vi "Check_Position_PN.vi"(0 "Visualisation only (no collision detection)":bool, 4 "Extrusion mode":bool, 5 "Collision mode":T1=enum."Traverse - All", 6 "Model Rotation (deg)":sgl[](array[numeric])=[0.0, 0.0, 0.0] format="%.2g", 7 "Traverse extruded position":sgl[](array[numeric])=[0.0, 0.0, 0.0] format="%.2g", 8 "Position to check":sgl[](array[numeric])=[0.0, 0.0, 0.0] format="%.2g", 9 "Traverse Name":string) -> (1 "Collision":bool, 3 "Error Comments":string)   [LabVIEW 2016]
uses:
  Collision_Detection/Triangles/EnFlo specific/Collision Mode.ctl
  <vilib>/Analysis/coordinate.llb/Euler Rotation Order.ctl
  <vilib>/Analysis/coordinate.llb/3D Cartesian Coordinate Rotation (Euler) (Scalar).vi
  <vilib>/Analysis/baseanly.llb/Unit Vector (DBL).vi
  <vilib>/Analysis/baseanly.llb/Real Dot Product.vi
  Globals/Constants_global.vi
  <vilib>/Analysis/NI_AALPro.lvlib
  <vilib>/Analysis/NI_AALBase.lvlib
panel:
  in  "3D graphics output":bool=TRUE
  # "X\n\nY\n\nZ"
  # "Roll\n\nPitch\n\nYaw"
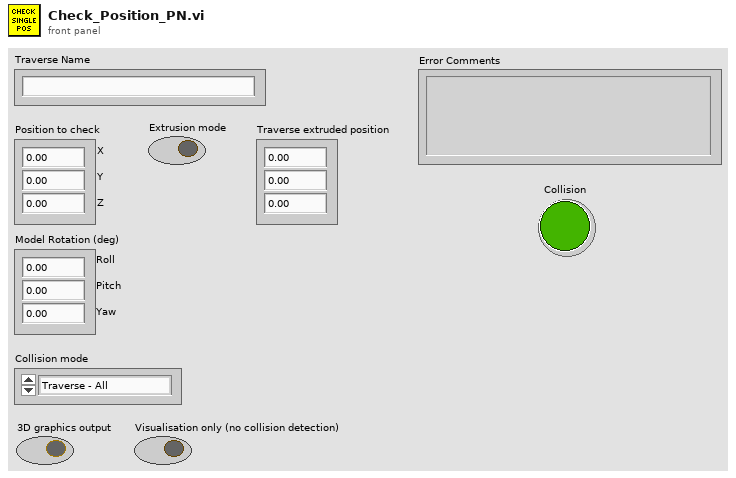
[diagram p1: front panel]
types:
  T1 = typedef "Collision Mode.ctl" = enum16{"Traverse - Tunnel", "Traverse - Model", "Traverse - Fixed objects", "Traverse - Traverse", "Traverse - All"}
  T2 = typedef "NI_AALPro.lvlib/Euler Rotation Order.ctl" = u16
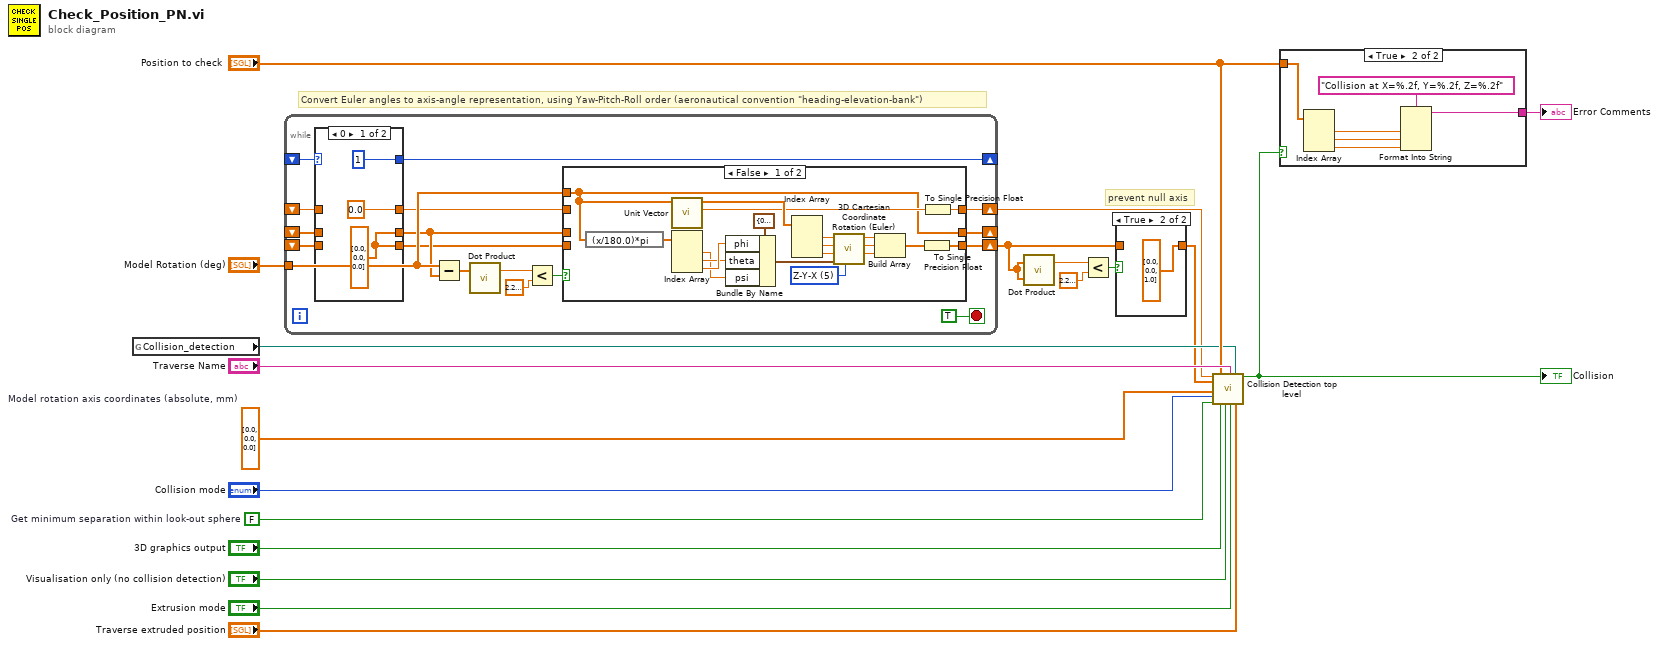
[diagram p0: block diagram]
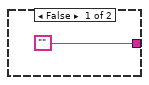
[diagram p5: hidden frame]
diagram:
  w10 = FALSE  # Get minimum separation within look-out sphere
  w19 = sgl[] [0.0, 0.0, 0.0]  # Model rotation axis coordinates (absolute, mm)
  # "prevent null axis"
  # "Convert Euler angles to axis-angle representation, using Yaw-Pitch-Roll order (aeronautical convention \"heading-elevation-bank\")"
  n1 = global read "Constants_global.vi" "Collision_detection"() -> (w14:path)
  n2 = while {
    shift-right: [w32] -> _
    shift-left: _ -> [w22]
    tunnel: "Model Rotation (deg)" -> [w33]
    shift-right: [w35] -> w2
    shift-left: _ -> [w20]
    shift-right: [w31] -> w6
    shift-left: _ -> [w24]
    shift-right: [w26] -> _
    shift-left: _ -> [w27]
    stop <- TRUE stop-if-true
    n3 = case shown="0" w27 {
      selector: w27 -> [_ w43]
      tunnel: [u8 1 w43] -> w26
      tunnel: [sgl 0.0 w42] -> w25
      tunnel: w24 -> [_ w42]
      tunnel: [w37 w41] -> w23
      tunnel: w22 -> [_ w41]
      tunnel: [w37 w40] -> w21
      tunnel: w20 -> [_ w40]
      frame 0 {
        w37 = sgl[] [0.0, 0.0, 0.0]
      }
      frame Default {
      }
    }
    n4 = Subtract(x=w33, y=w23) -> (x-y=w29:sgl[])
    n5 = call-poly <vilib>:"Dot Product.vi"("X Vector"=w29) -> ("X * Y"=w28:dbl)  [unwired: 1 in, 1 out]
    n6 = Less?(x=w28, y=2.220446049250313e-16) -> (x < y?=w30:bool)
    n7 = case shown="False" w30 {
      tunnel: w33 -> [w46 _]
      tunnel: w23 -> [_ w65]
      tunnel: [w45 w64] -> w35
      tunnel: [w46 w65] -> w32
      tunnel: w21 -> [_ w64]
      tunnel: [w44 w63] -> w31
      tunnel: w25 -> [_ w63]
      frame False {
        w49 = T2 5 items=["X-Y-Z", "X-Z-Y", "Y-X-Z", "Y-Z-X", "Z-X-Y", "Z-Y-X", "X-Y-X", "X-Z-X", "Y-X-Y", "Y-Z-Y", "Z-X-Z", "Z-Y-Z"] ("rotation order")
        n8 = expression code="(x/180.0)*pi" ("degrees to radians")(w46) -> (w54:sgl[])
        n9 = call-poly <vilib>:"Unit Vector.vi"("Input Vector"=w46) -> ("norm"=w47:dbl, "Unit Vector"=w59:dbl[])  [unwired: 8 in, 1 out]
        n10 = Index Array(array=w54) -> (element #1=w55:sgl, element #2=w56:sgl, element #3=w57:sgl)  [unwired: 3 in]
        n11 = Bundle By Name(cluster=cluster{"phi":dbl, "theta":dbl, "psi":dbl} {"phi"=0.0, "theta"=0.0, "psi"=0.0} ("Euler Angles"), "phi"=w57, "theta"=w56, "psi"=w55) -> (w58:cluster{"phi":dbl, "theta":dbl, "psi":dbl})
        n12 = Index Array(array=w59) -> (element #1=w62:dbl, element #2=w61:dbl, element #3=w60:dbl)  [unwired: 3 in]
        n13 = call-poly <vilib>:"3D Cartesian Coordinate Rotation (Euler).vi"("rotation order"=w49, "Euler Angles"=w58, "z"=w60, "y"=w61, "x"=w62) -> ("z out"=w52:dbl, "y out"=w51:dbl, "x out"=w50:dbl)  [unwired: 3 in, 1 out]
        n14 = Build Array(w50, w51, w52) -> (w48:dbl[])
        n15 = To Single Precision Float(number=w48) -> (single precision float=w45:sgl[])
        n16 = To Single Precision Float(number=w47) -> (single precision float=w44:sgl)
      }
      frame True {
      }
    }
  }
  n17 = call-poly <vilib>:"Dot Product.vi"("Y Vector"=w2, "X Vector"=w2) -> ("X * Y"=w5:dbl)  [unwired: 1 out]
  n18 = Less?(x=w5, y=2.220446049250313e-16) -> (x < y?=w3:bool)
  n19 = case shown="True" w3 {
    tunnel: w2 -> [w66 _]
    tunnel: [w66 sgl[] [0.0, 0.0, 1.0]] -> w1
    frame False {
    }
    frame True {
    }
  }
  n20 = call "Collision Detection top level.vi"("Model rotation (degrees)"=w6, "Model rotation axis (unit vector)"=w1, "Model rotation axis coordinates (absolute, mm)"=w19, "Collision mode"="Collision mode", "Get minimum separation within look-out sphere"=w10, "Traverse position (absolute, mm)"="Position to check", "3D graphics output"="3D graphics output", "Visualisation only (no collision detection)"="Visualisation only (no collision detection)", "Traverse name"="Traverse Name", "Extrusion mode"="Extrusion mode", "Rig geometry directory path"=w14, "Traverse extruded position"="Traverse extruded position") -> ("Collision"=w17:bool)  [unwired: 3 in, 4 out]
  "Collision" <- w17
  n21 = case shown="True" w17 {
    tunnel: "Position to check" -> [_ w74]
    tunnel: ["" w69] -> w15
    frame False {
    }
    frame True {
      n22 = Index Array(array=w74) -> (element #1=w73:sgl, element #2=w72:sgl, element #3=w71:sgl)  [unwired: 3 in]
      n23 = Format Into String(format string="Collision at X=%.2f, Y=%.2f, Z=%.2f", w73, w72, w71) -> (resulting string=w69:string)  [unwired: 2 in, 1 out]
    }
  }
  "Error Comments" <- w15
